vi "create.TradeBase.vi"(8 "error in (no error)":errorcluster, 11 "TradeBase in":refnum<class "TradeBase.lvclass">) -> (0 "error out":errorcluster, 3 "TradeBase out":refnum<class "TradeBase.lvclass">)   [LabVIEW 2020, in "TradeBase.lvclass"]
uses:
  TradeBase.lvclass
  FieldSpec.ctl
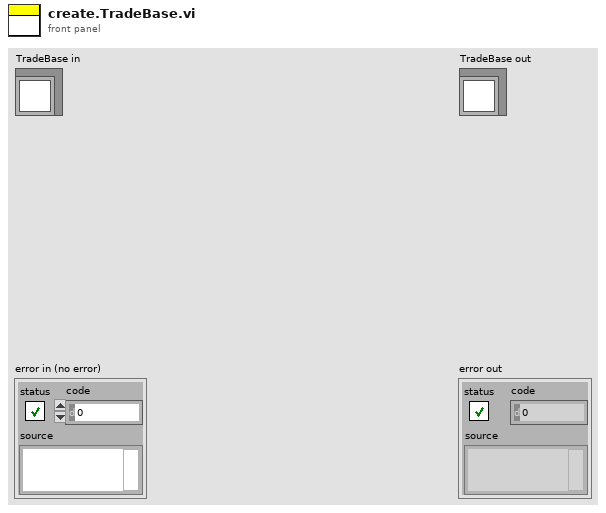
[diagram p1: front panel]
types:
  T1 = typedef "FieldSpec.ctl" = cluster{"Name":string, "Offset":i32, "Length":i32, "FieldType":enum16{"Alphanumeric", "Binary", "BinaryLongPrice", "BinaryShortPrice", "BitField", "PrintableAscii", "Value"}, "FieldValue":variant}
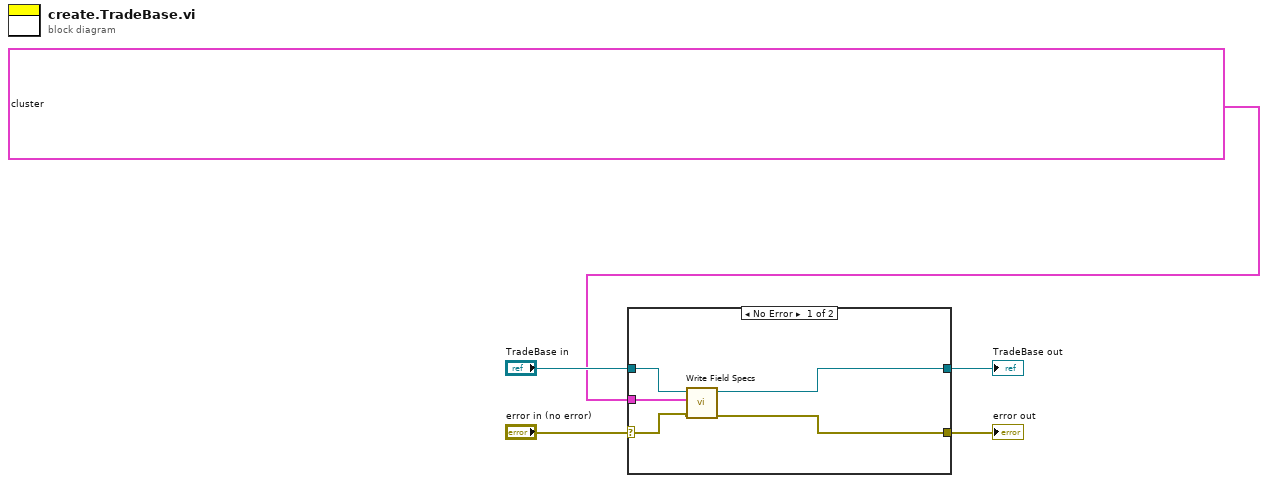
[diagram p0: block diagram]
diagram:
  n1 = case shown="No Error" "error in (no error)" {
    selector: "error in (no error)" -> [w8 w12]
    tunnel: [w7 w12] -> w4
    tunnel: [w6 w11] -> w2
    tunnel: "TradeBase in" -> [w10 w11]
    tunnel: T1[] [{"Name"="Length", "Offset"=0, "Length"=1, "FieldType"=enum."Binary", "FieldValue"=variant}, {"Name"="MessageType", "Offset"=1, "Length"=1, "FieldType"=enum."Value", "FieldValue"=variant}, {"Name"="Time Offset", "Offset"=2, "Length"=4, "FieldType"=enum."Binary", "FieldValue"=variant}, {"Name"="Order Id", "Offset"=6, "Length"=8, "FieldType"=enum."Binary", "FieldValue"=variant}, {"Name"="Side Indicator", "Offset"=14, "Length"=1, "FieldType"=enum."Alphanumeric", "FieldValue"=variant}, {"Name"="Quantity", "Offset"=15, "Length"=4, "FieldType"=enum."Binary", "FieldValue"=variant}, {"Name"="Symbol", "Offset"=19, "Length"=6, "FieldType"=enum."PrintableAscii", "FieldValue"=variant}, {"Name"="Price", "Offset"=25, "Length"=8, "FieldType"=enum."BinaryLongPrice", "FieldValue"=variant}, {"Name"="Execution Id", "Offset"=33, "Length"=8, "FieldType"=enum."PrintableAscii", "FieldValue"=variant}] ("appended array") -> [w9 _]
    frame No Error {
      n2 = call-dynamic "Write Field Specs.vi"("error in (no error)"=w8, "Field Specs"=w9, "MessageBase in"=w10) -> ("error out"=w7:errorcluster, "MessageBase out"=w6:refnum<class "TradeBase.lvclass">)  [unwired: 7 in]
    }
    frame Error {
    }
  }
  "error out" <- w4
  "TradeBase out" <- w2
